vi "AOMButtonControl.vi"(11 "AOM Ctrl":refnum<vi>) -> ()   [LabVIEW 2017]
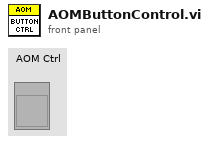
[diagram p1: front panel]
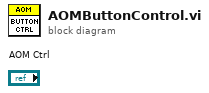
[diagram p0: block diagram]
diagram:
